vi "Send to Tulip.vi"(8 "Data file":string, 9 "Result":string, 11 "Serial number":string) -> (0 "error out":errorcluster, 1 "Status String":string, 3 "Response body":string)   [LabVIEW 2021]
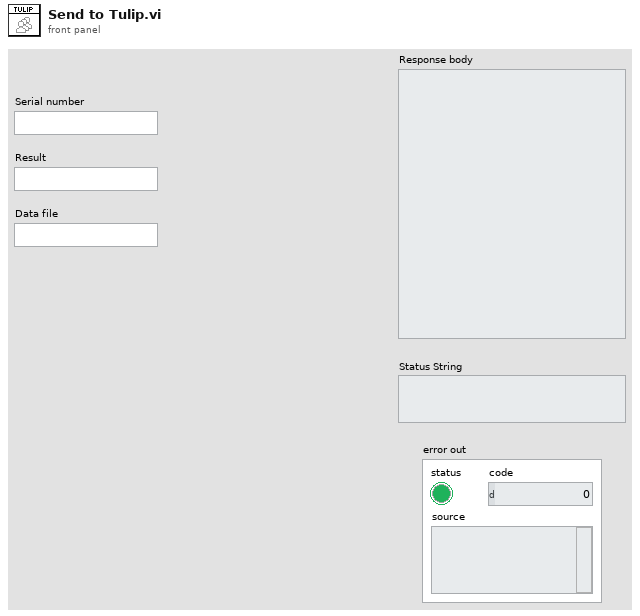
[diagram p1: front panel]
types:
  T1 = cluster{"id":string, "eujqt_serial_number":string, "ipmgv_parameter":string, "avnfl_result":string, "itjea_date":string, "rbhym_data_file":string}
  T2 = enum16{"Init", "Get headers", "Get", "Post", "Put", "Close"}
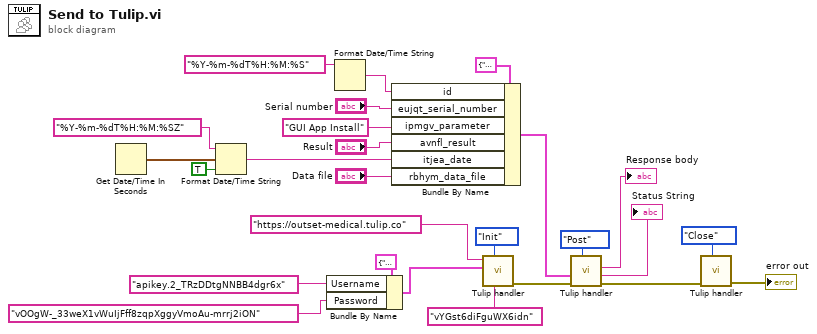
[diagram p0: block diagram]
diagram:
  n1 = Get Date/Time In Seconds() -> (seconds since 1Jan1904=w11:timestamp)
  n2 = Format Date/Time String(time format string (%c)="%Y-%m-%dT%H:%M:%SZ", seconds (now)=w11, UTC format=TRUE) -> (date/time string=w9:string)
  n3 = Bundle By Name(cluster=cluster{"Username":string, "Password":string} {"Username"="apikey.2_WNWgDzkcRL7LwQrSC", "Password"="uUTRYqQF2kxie-OG2NdFiDN_Ok5rwnamrdCqWvd0OVz"} ("Authentication"), "Username"="apikey.2_TRzDDtgNNBB4dgr6x", "Password"="vOOgW-_33weX1vWuIjFff8zqpXggyVmoAu-mrrj2iON") -> (w23:cluster{"Username":string, "Password":string})
  n4 = Format Date/Time String(time format string (%c)="%Y-%m-%dT%H:%M:%S") -> (date/time string=w5:string)  [unwired: 2 in]
  n5 = Bundle By Name(cluster=T1 {"id"="", "eujqt_serial_number"="", "ipmgv_parameter"="", "avnfl_result"="", "itjea_date"="", "rbhym_data_file"=""} ("Body"), "id"=w5, "eujqt_serial_number"="Serial number", "ipmgv_parameter"="GUI App Install", "avnfl_result"="Result", "itjea_date"=w9, "rbhym_data_file"="Data file") -> (w4:T1)
  n6 = call "Tulip handler.vi"("Table ID"="vYGst6diFguWX6idn", "State"=T2."Init", "Authentication"=w23, "URL"="https://outset-medical.tulip.co") -> ("error out"=w26:errorcluster)  [unwired: 5 in, 2 out]
  n7 = call "Tulip handler.vi"("State"=T2."Post", "error in"=w26, "Body"=w4) -> ("error out"=w17:errorcluster, "Status String"=→"Status String":string, "Response body"=→"Response body":string)  [unwired: 6 in]
  n8 = call "Tulip handler.vi"("State"=T2."Close", "error in"=w17) -> ("error out"=→"error out":errorcluster)  [unwired: 7 in, 2 out]
